vi "Handle Event.vi"(6 "Action in":T2, 7 "Data in":path, 9 "Event Cluster":T3, 10 "Container State":T1, 11 "Path Selector in":refnum<class "MGI Path Selector.lvclass">) -> (1 "Discard?":bool, 2 "Facade complete?":bool, 3 "Path Selector out":refnum<class "MGI Path Selector.lvclass">, 4 "Action out":T2, 5 "Data out":path)   [LabVIEW 2020, in "MGI Path Selector.lvclass"]
doc: "This VI is called by every event in the XControl's facade VI. It Handles the Event Cluster type as appropriate.\n\nAuthored by Shawn Walpole\nsupport@mooregoodideas.com\nwww.mooregoodideas.com\n\nCopyright (c) 2013, Moore Good Ideas, Inc.\n\nAll rights reserved.\n\nRedistribution and use in source and binary forms, with or without modification, are permitted provided that the following conditions are met:\n\n * Redistributions of source code must retain the above copyright notice, this list of conditions and the following disclaimer.\n * Redistributions in binary form must reproduce the above copyright notice, this list of conditions and the following disclaimer in the documentation and/or other materials provided with the distribution.\n * Neither the name of Moore Good Ideas, Inc. nor the names of its contributors may be used to endorse or promote products derived from this software without specific prior written permission.\n\nTHIS SOFTWARE IS PROVIDED BY THE COPYRIGHT HOLDERS AND CONTRIBUTORS \"AS IS\" AND ANY EXPRESS OR IMPLIED WARRANTIES, INCLUDING, BUT NOT LIMITED TO, THE IMPLIED WARRANTIES OF MERCHANTABILITY AND FITNESS FOR A PARTICULAR PURPOSE ARE DISCLAIMED. IN NO EVENT SHALL THE COPYRIGHT OWNER OR CONTRIBUTORS BE LIABLE FOR ANY DIRECT, INDIRECT, INCIDENTAL, SPECIAL, EXEMPLARY, OR CONSEQUENTIAL DAMAGES (INCLUDING, BUT NOT LIMITED TO, PROCUREMENT OF SUBSTITUTE GOODS OR SERVICES; LOSS OF USE, DATA, OR PROFITS; OR BUSINESS INTERRUPTION) HOWEVER CAUSED AND ON ANY THEORY OF LIABILITY, WHETHER IN CONTRACT, STRICT LIABILITY, OR TORT (INCLUDING NEGLIGENCE OR OTHERWISE) ARISING IN ANY WAY OUT OF THE USE OF THIS SOFTWARE, EVEN IF ADVISED OF THE POSSIBILITY OF SUCH DAMAGE."
uses:
  <userlib>/_MGI/User Interface/Path Selector XControl/Class Hierarchy/MGI Path Selector.lvclass
  <userlib>/_MGI/User Interface/Path Selector XControl/Event Cluster.ctl
  <vilib>/event_ctls.llb/lveventtype.ctl
  <vilib>/Utility/miscctls.llb/LVPoint32TypeDef.ctl
  <vilib>/_xctls/Action.ctl
  <vilib>/_xctls/Container State.ctl
  <userlib>/_MGI/User Interface/Path Selector XControl/Class Hierarchy/MGI Path Selector.lvclass/MGI Path Selector.ctl
  <vilib>/_xctls/XControlSupport.lvlib
  <userlib>/_MGI/User Interface/Path Selector XControl/MGI Path Selector.xctl
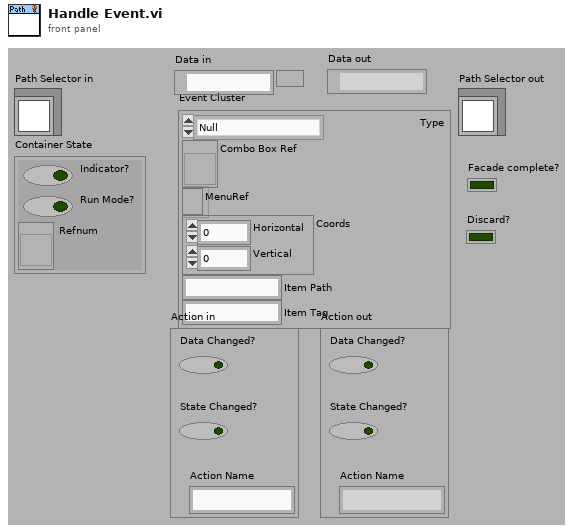
[diagram p1: front panel]
types:
  T1 = typedef "XControlSupport.lvlib/Container State.ctl" = cluster{"Indicator?":bool, "Run Mode?":bool, " Refnum":refnum<vi>}
  T2 = typedef "XControlSupport.lvlib/Action.ctl" = cluster{"Data Changed?":bool, "State Changed?":bool, "Action Name":string}
  T3 = typedef "MGI Path Selector.xctl/Event Cluster.ctl" = cluster{"Type":T4, "Combo Box Ref":refnum<vi>, "MenuRef":refnum<k9>, "Coords":T5, "Item Path":string, "Item Tag":string}
  T4 = typedef "lveventtype.ctl" = enum32{"Null", "Timeout", "Annotation Menu Selection", "Annotation Menu Selection?", "App Instance Close", "App Instance Close?", "Autoscale Range Change", "Bookmark Info Change", "Cell Edit", "Cell Edit?", "Cursor Grab", "Cursor Grab?", "Cursor Menu Selection", "Cursor Menu Selection?", "Cursor Move", "Cursor Release", "Data Change", "Direction Change", "Display State Change", "Drag Ended", "Drag Enter", "Drag Leave", "Drag Over", "Drag Source Update", "Drag Starting", "Drag Starting?", "Drop", "Exec State Change", "Key Down", "Key Down?", "Key Repeat", "Key Repeat?", "Key Up", "Listbox Double Click", "Menu Activation?", "Menu Selection (App)", "Menu Selection? (App)", "Menu Selection (User)", "Mouse Down", "Mouse Down?", "Mouse Enter", "Mouse Leave", "Mouse Move", "Mouse Up", "Mouse Wheel", "NI Security User Change (App)", "Pane Size", "Panel Close", "Panel Close?", "Panel Resize", "Plot Attribute Change", "Scale Range Change", "Shortcut Menu Activation?", "Shortcut Menu Selection (App)", "Shortcut Menu Selection? (App)", "Shortcut Menu Selection (User)", "Tree Double Click", "Tree Drag", "Tree Drag?", "Tree Drop", "Tree Drop?", "Tree Item Close", "Tree Item Close?", "Tree Item Open", "Tree Item Open?", "User Event", "Value Change"}
  T5 = typedef "LVPoint32TypeDef.ctl" = cluster{"Horizontal":i32, "Vertical":i32}
  T6 = typedef "LVRectTypeDef.ctl" = cluster{"Left":i16, "Top":i16, "Right":i16, "Bottom":i16}
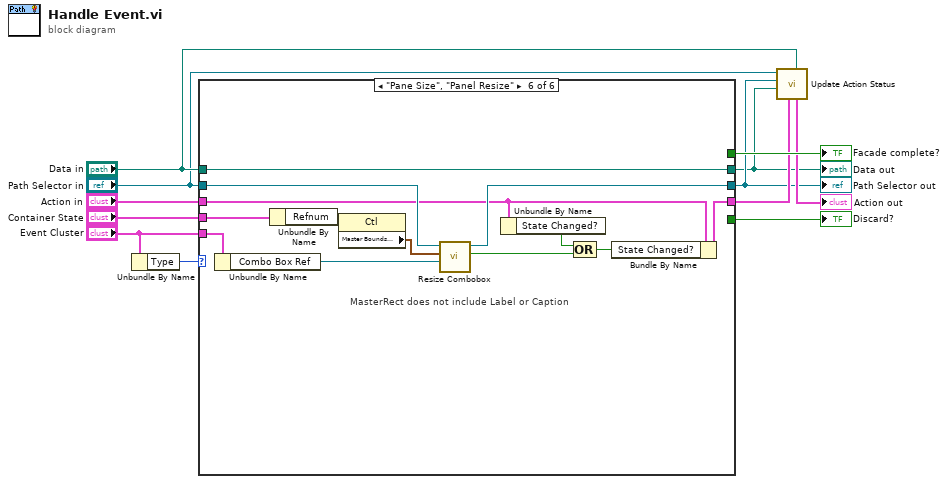
[diagram p0: block diagram]
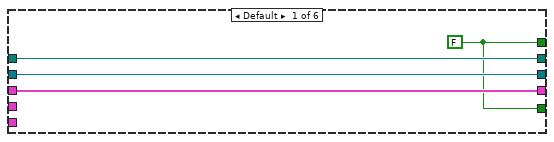
[diagram p2: hidden frame]
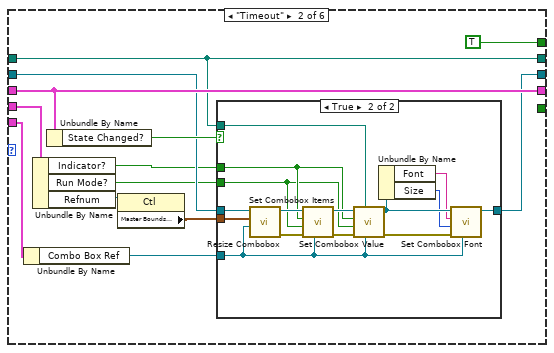
[diagram p3: hidden frame]
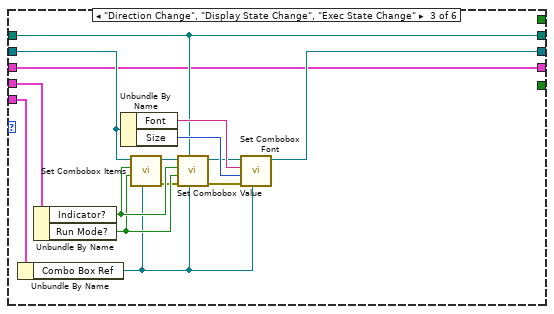
[diagram p5: hidden frame]
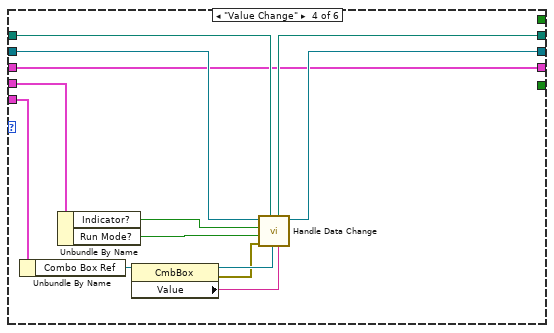
[diagram p6: hidden frame]
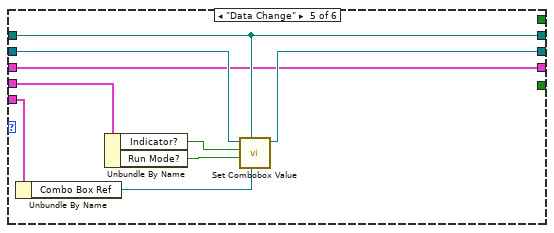
[diagram p7: hidden frame]
diagram:
  n1 = Unbundle By Name("Event Cluster") -> ("Type"=w12:T4)
  n2 = case shown="\"Pane Size\", \"Panel Resize\"" w12 {
    tunnel: "Path Selector in" -> [w16 w21 w56 w65 w80 w88]
    tunnel: [w16 w20 w55 w64 w81 w87] -> w2
    tunnel: "Data in" -> [w15 w17 w47 w63 w82 w94]
    tunnel: [w13 TRUE _ _ _ _] -> w11
    tunnel: [w15 w17 w47 w62 w82 w94] -> w1
    tunnel: "Container State" -> [_ w26 w60 w67 w77 w92]
    tunnel: "Action in" -> [w14 w28 w46 w61 w74 w86]
    tunnel: "Event Cluster" -> [_ w24 w59 w73 w79 w95]
    tunnel: [w14 w28 w46 w61 w74 w93] -> w5
    tunnel: [w13 _ _ _ _ _] -> w7
    frame Default {
      w13 = FALSE
    }
    frame "Timeout" {
      n3 = Unbundle By Name(w24) -> ("Combo Box Ref"=w23:refnum<vi>)
      n4 = Unbundle By Name(w26) -> ("Indicator?"=w19:bool, "Run Mode?"=w18:bool, "Refnum"=w27:refnum<vi>)
      n5 = Unbundle By Name(w28) -> ("State Changed?"=w22:bool)
      n6 = property on="Property Node" class="Ctl"(reference=w27) -> ("Master Bounds Rect"=w25:T6)  [unwired: 1 in, 2 out]
      n7 = case shown="True" w22 {
        tunnel: w25 -> [_ w45]
        tunnel: w23 -> [_ w38]
        tunnel: w21 -> [w30 w44]
        tunnel: [w30 w37] -> w20
        tunnel: w19 -> [_ w36]
        tunnel: w18 -> [_ w35]
        tunnel: w17 -> [_ w34]
        frame False {
        }
        frame True {
          n8 = call-dynamic "Resize Combobox.vi"("Cmb Box"=w38, "Bounds"=w45, "Path Selector in"=w44) -> ("error out"=w41:errorcluster, "Path Selector out"=w42:refnum<class "MGI Path Selector.lvclass">)  [unwired: 6 in, 1 out]
          n9 = call-dynamic "Set Combobox Items.vi"("Combo Box Ref"=w38, "error in (no error)"=w41, "Run Mode?"=w35, "Indicator?"=w36, "Path Selector in"=w42) -> ("error out"=w40:errorcluster, "Path Selector out"=w43:refnum<class "MGI Path Selector.lvclass">)  [unwired: 4 in, 1 out]
          n10 = call-dynamic "Set Combobox Value.vi"("Combo Box Ref"=w38, "Data"=w34, "error in (no error)"=w40, "Run Mode?"=w35, "Indicator?"=w36, "Path Selector in"=w43) -> ("error out"=w39:errorcluster, "Path Selector out"=w33:refnum<class "MGI Path Selector.lvclass">)  [unwired: 4 in]
          n11 = Unbundle By Name(w33) -> ("Font"=w31:string, "Size"=w32:i32)
          n12 = call-dynamic "Set Combobox Font.vi"("Combo Box Ref"=w38, "error in (no error)"=w39, "Font Size (0: No Change)"=w32, "Font (\"\": No Change)"=w31, "Path Selector in"=w33) -> ("Path Selector out"=w37:refnum<class "MGI Path Selector.lvclass">)  [unwired: 5 in, 1 out]
        }
      }
    }
    frame "Direction Change", "Display State Change", "Exec State Change" {
      n13 = Unbundle By Name(w59) -> ("Combo Box Ref"=w52:refnum<vi>)
      n14 = Unbundle By Name(w60) -> ("Indicator?"=w54:bool, "Run Mode?"=w53:bool)
      n15 = Unbundle By Name(w56) -> ("Font"=w57:string, "Size"=w58:i32)
      n16 = call-dynamic "Set Combobox Items.vi"("Combo Box Ref"=w52, "Run Mode?"=w53, "Indicator?"=w54, "Path Selector in"=w56) -> ("error out"=w49:errorcluster, "Path Selector out"=w51:refnum<class "MGI Path Selector.lvclass">)  [unwired: 5 in, 1 out]
      n17 = call-dynamic "Set Combobox Value.vi"("Combo Box Ref"=w52, "Data"=w47, "error in (no error)"=w49, "Run Mode?"=w53, "Indicator?"=w54, "Path Selector in"=w51) -> ("error out"=w48:errorcluster, "Path Selector out"=w50:refnum<class "MGI Path Selector.lvclass">)  [unwired: 4 in]
      n18 = call-dynamic "Set Combobox Font.vi"("Combo Box Ref"=w52, "error in (no error)"=w48, "Font Size (0: No Change)"=w58, "Font (\"\": No Change)"=w57, "Path Selector in"=w50) -> ("Path Selector out"=w55:refnum<class "MGI Path Selector.lvclass">)  [unwired: 5 in, 1 out]
    }
    frame "Value Change" {
      n19 = Unbundle By Name(w73) -> ("Combo Box Ref"=w72:refnum<vi>)
      n20 = Unbundle By Name(w67) -> ("Indicator?"=w68:bool, "Run Mode?"=w66:bool)
      n21 = property class="CmbBox"(reference=w72) -> (reference out=w70:refnum<vi>, error out=w69:errorcluster, "Value"=w71:string)  [unwired: 1 in]
      n22 = call-dynamic "Handle Data Change.vi"("Value"=w71, "Combo Box Ref"=w70, "Data in"=w63, "error in (no error)"=w69, "Run Mode?"=w66, "Indicator?"=w68, "Path Selector in"=w65) -> ("Path Selector out"=w64:refnum<class "MGI Path Selector.lvclass">, "Data out"=w62:path)  [unwired: 2 in, 1 out]
    }
    frame "Data Change" {
      n23 = Unbundle By Name(w79) -> ("Combo Box Ref"=w78:refnum<vi>)
      n24 = Unbundle By Name(w77) -> ("Indicator?"=w75:bool, "Run Mode?"=w76:bool)
      n25 = call-dynamic "Set Combobox Value.vi"("Combo Box Ref"=w78, "Data"=w82, "Run Mode?"=w76, "Indicator?"=w75, "Path Selector in"=w80) -> ("Path Selector out"=w81:refnum<class "MGI Path Selector.lvclass">)  [unwired: 5 in, 1 out]
    }
    frame "Pane Size", "Panel Resize" {
      # "MasterRect does not include Label or Caption"
      n26 = Unbundle By Name(w95) -> ("Combo Box Ref"=w90:refnum<vi>)
      n27 = Unbundle By Name(w92) -> ("Refnum"=w91:refnum<vi>)
      n28 = property on="Property Node" class="Ctl"(reference=w91) -> ("Master Bounds Rect"=w89:T6)  [unwired: 1 in, 2 out]
      n29 = call-dynamic "Resize Combobox.vi"("Cmb Box"=w90, "Bounds"=w89, "Path Selector in"=w88) -> ("Changed?"=w85:bool, "Path Selector out"=w87:refnum<class "MGI Path Selector.lvclass">)  [unwired: 6 in, 1 out]
      n30 = Unbundle By Name(w86) -> ("State Changed?"=w84:bool)
      n31 = Compound Arithmetic op=OR(w84, w85) -> (w83:bool)
      n32 = Bundle By Name(cluster=w86, "State Changed?"=w83) -> (w93:T2)
    }
  }
  "Path Selector out" <- w2
  "Data out" <- w1
  "Facade complete?" <- w11
  "Discard?" <- w7
  n33 = call-dynamic "Update Action Status.vi"("Data (orig)"="Data in", "Action in"=w5, "Data"=w1, "Path Selector"=w2, "Path Selector (orig)"="Path Selector in") -> ("Action out"=→"Action out":T2)  [unwired: 5 in, 1 out]
